vi "My_DHT11_Labview1_Gweb2.vi"() -> ()   [LabVIEW 2024]
uses:
  <vilib>/Instr/_visa.llb/VISA Configure Serial Port (Instr).vi
  GlobalTempHum.vi
panel:
  out "read buffer":string
  in  "?":bool
  in  "VISA Arduino Uno":refnum<visa-resource-name>
  # "Environmental Control System for Greenhouses\n\nMonitoring System"
  # "House No. 1"
  # "Eng. Yahia Gaddal\ngaddal18@gmail.com"
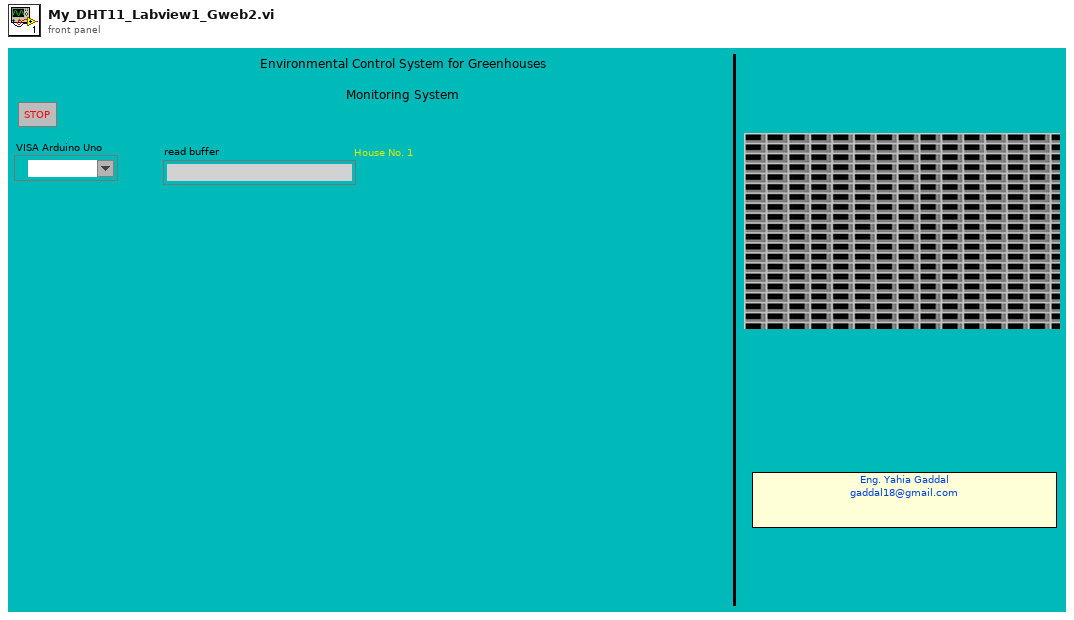
[diagram p1: front panel]
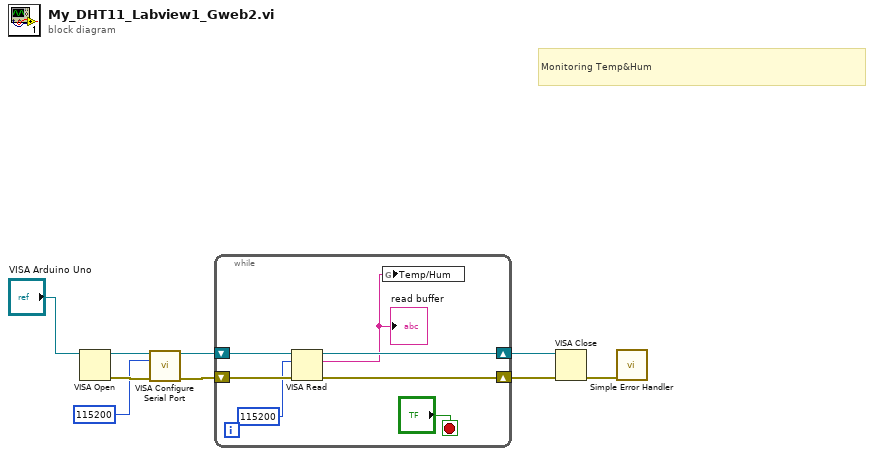
[diagram p0: block diagram]
diagram:
  # "Monitoring Temp&Hum"
  n1 = VISA Open(VISA resource name="VISA Arduino Uno") -> (VISA resource name=w9:refnum<visa-resource-name>, error out=w8:errorcluster)  [unwired: 4 in]
  n2 = call-poly "VISA Configure Serial Port"("VISA resource name"=w9, "baud rate (9600)"=u32 115200, "error in (no error)"=w8) -> ("VISA resource name out"=w7:refnum<visa-resource-name>, "error out"=w6:errorcluster)  [unwired: 11 in]
  n3 = while {
    shift-right: [w13] -> w5
    shift-left: w7 -> [w16]
    shift-right: [w12] -> w4
    shift-left: w6 -> [w15]
    stop <- "?" stop-if-true
    n4 = VISA Read(VISA resource name=w16, byte count=u32 115200, error in (no error)=w15) -> (VISA resource name out=w13:refnum<visa-resource-name>, read buffer=w10:string, error out=w12:errorcluster)  [unwired: 1 out]
    "read buffer" <- w10
    n5 = global write "GlobalTempHum.vi" "Temp/Hum"(w10) -> ()
  }
  n6 = VISA Close(VISA resource name=w5, error in (no error)=w4) -> (error out=w1:errorcluster)
  n7 = call <vilib>:"Simple Error Handler.vi"("error in (no error)"=w1) -> ()  [unwired: 4 in, 5 out]
